vi "Graph_Server_RegExp (SubVI).vi"(6 "regular expression":string, 8 "Error In":errorcluster, 11 "command":string) -> (0 "Error Out":errorcluster, 2 "trimmed string":string, 3 "trimmed string 2":string)   [LabVIEW 2018]
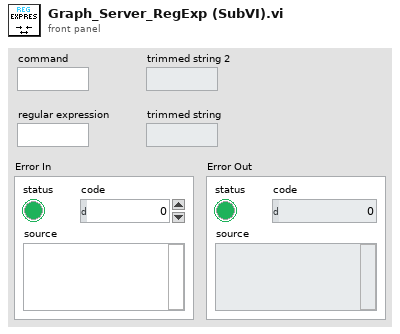
[diagram p1: front panel]
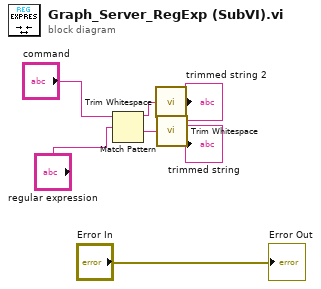
[diagram p0: block diagram]
diagram:
  n1 = Match Pattern(string="command", regular expression="regular expression") -> (before substring=w4:string, after substring=w2:string)  [unwired: 1 in, 2 out]
  n2 = call <vilib>:"Trim Whitespace.vi"("string"=w4) -> ("trimmed string"=→"trimmed string 2":string)  [unwired: 1 in]
  n3 = call <vilib>:"Trim Whitespace.vi"("string"=w2) -> ("trimmed string"=→"trimmed string":string)  [unwired: 1 in]
  "Error Out" <- "Error In"
